vi "Refname to String (Sensor).vi"(1 "Sensor Refname":T1) -> (0 "Refnum Name":string)   [LabVIEW 2015, in "Sprocket.lvlib"]
uses:
  lib/Sprocket.lvlib
  Refname Enum (Sensor).ctl
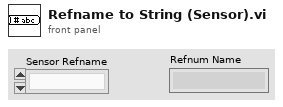
[diagram p1: front panel]
types:
  T1 = typedef "Sprocket.lvlib/Refname Enum (Sensor).ctl" = enum16{""}
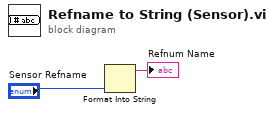
[diagram p0: block diagram]
diagram:
  n1 = Format Into String("Sensor Refname") -> (resulting string=→"Refnum Name":string)  [unwired: 3 in, 1 out]
